vi "MAP_SubVI.vi"(0 "High Byte":u8, 3 "Low Byte":u8) -> (7 "MAP":dbl)   [LabVIEW 2012]
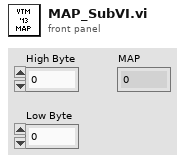
[diagram p1: front panel]
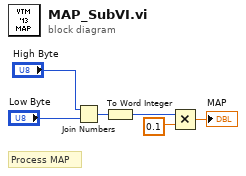
[diagram p0: block diagram]
diagram:
  # "Process MAP"
  n1 = Join Numbers(hi="High Byte", lo="Low Byte") -> ((hi.lo)=w4:u16)
  n2 = To Word Integer(number=w4) -> (16bit integer=w5:i16)
  n3 = Multiply(x=w5, y=0.1) -> (x*y=→"MAP":dbl)
